vi "CredentialCheck.vi"(10 "User Creds":T1) -> (1 "Access":u16, 2 "Name":string, 3 "Badge Num":string)   [LabVIEW 2023]
uses:
  UserCredentials.ctl
  <vilib>/Utility/miscctls.llb/LVSelectionTypeDef.ctl
panel:
  in  "Close Button":bool
  out "OK":bool
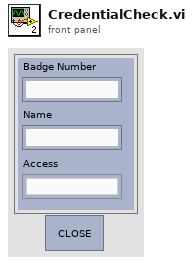
[diagram p1: front panel]
types:
  T1 = typedef "UserCredentials.ctl" = cluster{"Badge Number":string, "Name":string, "Access":enum16{"", "Operator", "Admin", "Engineer"}}
  T2 = typedef "LVSelectionTypeDef.ctl" = cluster{"Selection Start":u32, "Selection End":u32}
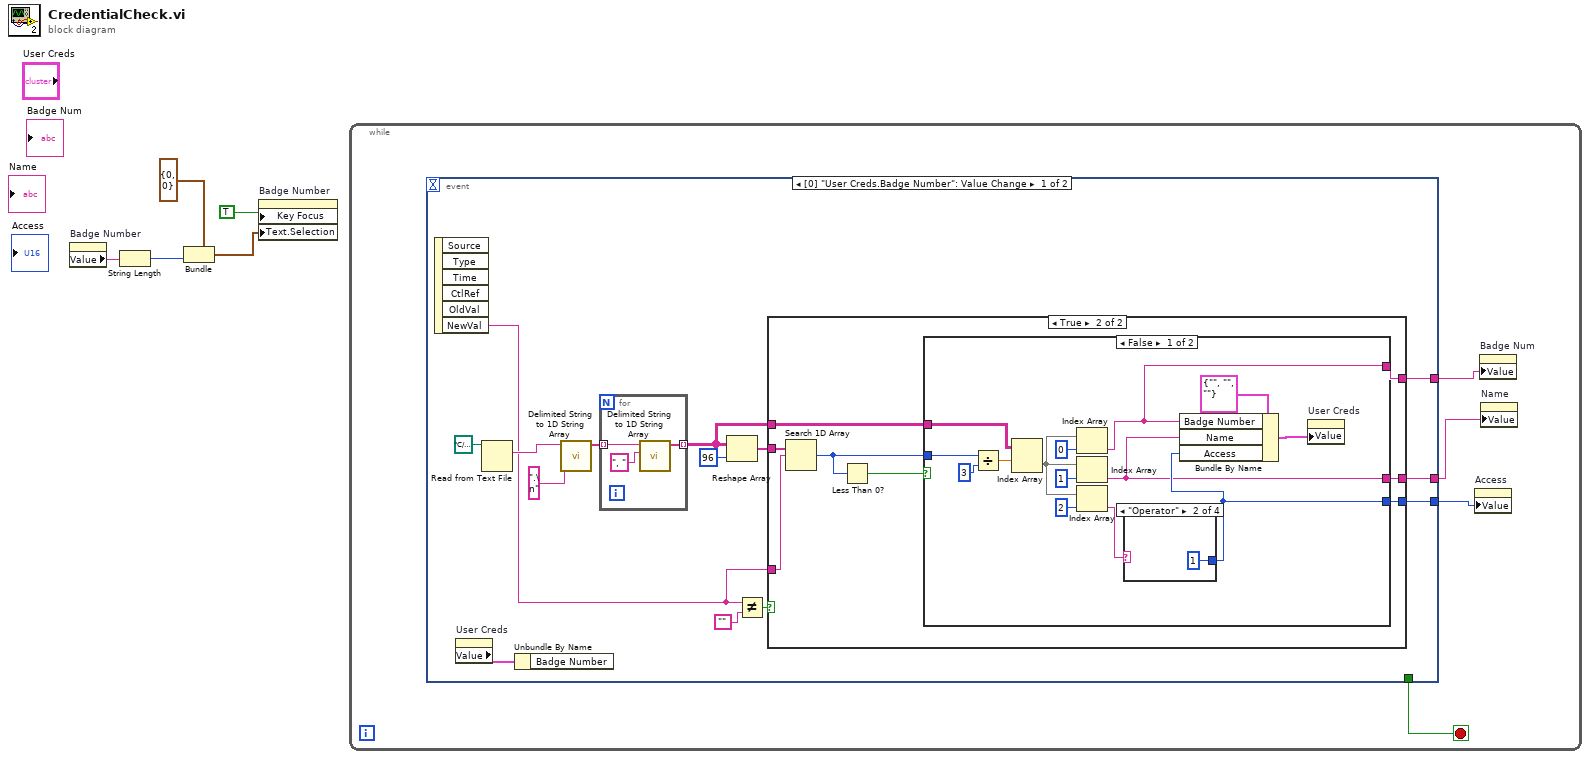
[diagram p0: block diagram]
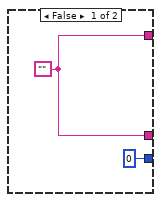
[diagram p2: hidden frame]
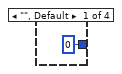
[diagram p3: hidden frame]
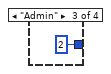
[diagram p4: hidden frame]
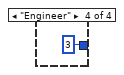
[diagram p5: hidden frame]
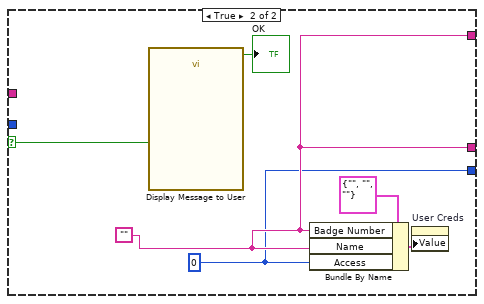
[diagram p6: hidden frame]
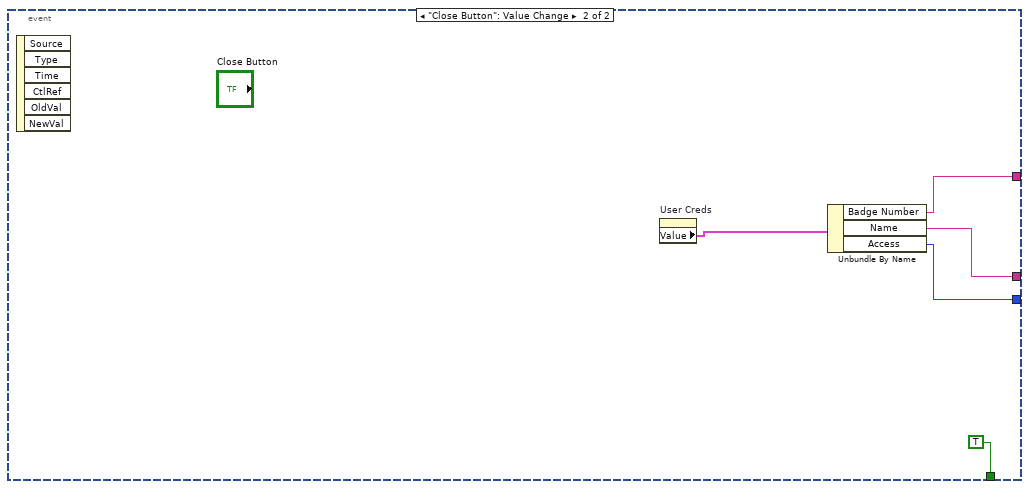
[diagram p7: hidden frame]
diagram:
  n1 = property on="Badge Number" class="Str"() -> ("Value"=w1:string)  [unwired: 2 in, 2 out]
  n2 = String Length(string=w1) -> (length=w3:i32)
  n3 = Bundle(cluster=T2 {"Selection Start"=0, "Selection End"=0} ("Text.Selection"), "Selection End"=w3) -> (w4:T2)  [unwired: 1 in]
  n4 = property on="Badge Number" class="Str"("Key Focus"=TRUE, "Text.Selection"=w4) -> ()  [unwired: 2 in, 2 out]
  n5 = while {
    stop <- w9 stop-if-true
    n6 = event shown="[0] \"User Creds.Badge Number\": Value Change" {
      selector: _ -> [_ _]
      dyn-events: _ -> [_ _]
      timeout: _ -> [_ _]
      tunnel: [_ TRUE] -> w9
      tunnel: [w12 w62] -> w6
      tunnel: [w11 w63] -> w7
      tunnel: [w10 w64] -> w8
      event Value Change {
        n7 = event-data() -> ("NewVal"=w13:string)  [unwired: 1 in, 5 out]
        n8 = property on="User Creds" class="Clust (strict)"() -> ("Value"=w23:T1)  [unwired: 2 in, 2 out]
        n9 = Read from Text File(file (use dialog)=path "C:/Users/Public/Documents/Grid2093/Security/Permissions.txt") -> (text=w18:string)  [unwired: 3 in, 3 out]
        n10 = Unbundle By Name(w23) -> ()  [unwired: 1 out]
        n11 = call <vilib>:"Delimited String to 1D String Array.vi"("delimiter"=".\n", "delimited string"=w18) -> ("string array"=w19:string[])  [unwired: 9 in]
        n12 = for {
          tunnel: w19 -> [w60] mode=indexing
          tunnel: [w58] -> w21 mode=indexing
          n13 = call <vilib>:"Delimited String to 1D String Array.vi"("delimiter"=", ", "delimited string"=w60) -> ("string array"=w58:string[])  [unwired: 9 in]
        }
        n14 = Reshape Array(w21, 96 ("dimension size")) -> (w20:string[])
        n15 = Not Equal?(x=w13, y="") -> (x != y?=w22:bool)
        n16 = case shown="True" w22 {
          tunnel: w20 -> [_ w33]
          tunnel: w21 -> [_ w30]
          tunnel: w13 -> [_ w29]
          tunnel: [u16 0 ("Access") w28] -> w12
          tunnel: [w25 w27] -> w11
          tunnel: [w25 w26] -> w10
          frame False {
            w25 = ""
          }
          frame True {
            n17 = Search 1D Array(1D array=w33, element=w29) -> (index of element=w31:i32)  [unwired: 1 in]
            n18 = Less Than 0?(x=w31) -> (x < 0?=w32:bool)
            n19 = case shown="False" w32 {
              selector: w32 -> [_ w57]
              tunnel: w31 -> [w47 _]
              tunnel: w30 -> [w44 _]
              tunnel: [w36 w52] -> w28
              tunnel: [w35 w53] -> w27
              tunnel: [w34 w53] -> w26
              frame False {
                n20 = Divide(x=w47, y=3) -> (x/y=w45:dbl)
                n21 = Index Array(array=w44, index (row)=w45) -> (element=w40:string[])  [unwired: 1 in]
                n22 = Index Array(array=w40, index=0) -> (element=w34:string)
                n23 = Index Array(array=w40, index=1) -> (element=w35:string)
                n24 = Index Array(array=w40, index=2) -> (element=w37:string)
                n25 = case shown="\"Operator\"" w37 {
                  tunnel: [u16 0 ("Access") u16 1 ("Access") u16 2 ("Access") u16 3 ("Access")] -> w36
                  frame "", Default {
                  }
                  frame "Operator" {
                  }
                  frame "Admin" {
                  }
                  frame "Engineer" {
                  }
                }
                n26 = Bundle By Name(cluster=T1 {"Badge Number"="", "Name"="", "Access"=enum.""} ("User Creds"), "Badge Number"=w34, "Name"=w35, "Access"=w36) -> (w38:T1)
                n27 = property on="User Creds" class="Clust (strict)"("Value"=w38) -> ()  [unwired: 2 in, 2 out]
              }
              frame True {
                w52 = u16 0 ("Access")
                w53 = ""
                n28 = call "Display Message to User"("Enable"=w57) -> ("OK"=→"OK":bool)  [unwired: 9 in, 1 out]
                n29 = Bundle By Name(cluster=T1 {"Badge Number"="", "Name"="", "Access"=enum.""} ("User Creds"), "Badge Number"=w53, "Name"=w53, "Access"=w52) -> (w54:T1)
                n30 = property on="User Creds" class="Clust (strict)"("Value"=w54) -> ()  [unwired: 2 in, 2 out]
              }
            }
          }
        }
      }
      event "Close Button": Value Change {
        n31 = event-data() -> ()  [unwired: 1 in, 6 out]
        n32 = property on="User Creds" class="Clust (strict)"() -> ("Value"=w61:T1)  [unwired: 2 in, 2 out]
        n33 = Unbundle By Name(w61) -> ("Badge Number"=w64:string, "Name"=w63:string, "Access"=w62:enum16{"", "Operator", "Admin", "Engineer"})
      }
    }
    n34 = property on="Access" class="DigNum (strict)"("Value"=w6) -> ()  [unwired: 2 in, 2 out]
    n35 = property on="Badge Num" class="Str"("Value"=w8) -> ()  [unwired: 2 in, 2 out]
    n36 = property on="Name" class="Str"("Value"=w7) -> ()  [unwired: 2 in, 2 out]
  }
